vi "Process.vi"(8 "error in":errorcluster, 11 "SMO.EmbeddedUI":refnum<class "Embedded UI.BasicTemplate.lvclass">) -> (0 "error out":errorcluster, 3 "SMO.EmbeddedUI out":refnum<class "Embedded UI.BasicTemplate.lvclass">)   [LabVIEW 2019, in "Embedded UI.BasicTemplate.lvclass"]
doc: "---------------------------------------------------------------\nJKI State Machine Objects™\nhttp://jki.net/state-machine-objects/\nCopyright (C) 2005-2015, JKI <info@jki.net>\nALL RIGHTS RESERVED"
uses:
  Embedded UI.BasicTemplate.lvclass
  C:/Program Files (x86)/National Instruments/LabVIEW 2019/vi.lib/JKI/JKI SMO/SMO/SMO.lvclass
  C:/Users/patrick/Documents/GitHub/Embedded-SMO/lvsrc/SMO.UI.Embedded/SMO.UI.Embedded.lvclass
  <vilib>/JKI/JKI SMO/SMO/Typedefs/Parent Call--Enum.ctl
  <vilib>/JKI/JKI SMO/SMO/SMO.lvclass/SMO.ctl
  Embedded UI/Typedefs/UI State.ctl
  <vilib>/JKI/JKI SMO/SMO/Private/ReftoDVR--SMO.vi
  Embedded UI/Embedded UI.lvclass
  <vilib>/JKI/JKI SMO/SMO/SMO.lvclass
  C:/Users/patrick/Documents/GitHub/Embedded-SMO/lvsrc/SMO.UI.Embedded/Embedded UI.lvclass
  C:/Program Files (x86)/National Instruments/LabVIEW 2019/vi.lib/JKI/JKI SMO/SMO.UI/SMO.UI.lvclass
panel:
  # "Embedded UI SMO\nJoseph Albro,\nLevylab\nUniversity of Pittsburgh\n\nImportant:\nKeep all of the information you want displayed inside this box."
  # "For instructions on how to use the JKI State Machine Objects, examples and video tutorials, visit:\nhttp://jki.net/state-machine-objects/\n\nJKI State Machine Objects™\nhttp://jki.net/state-machine-objects/\nCopyright (C) 2005-2015, JKI <info@jki.net>\nALL RIGHTS RESERVED"
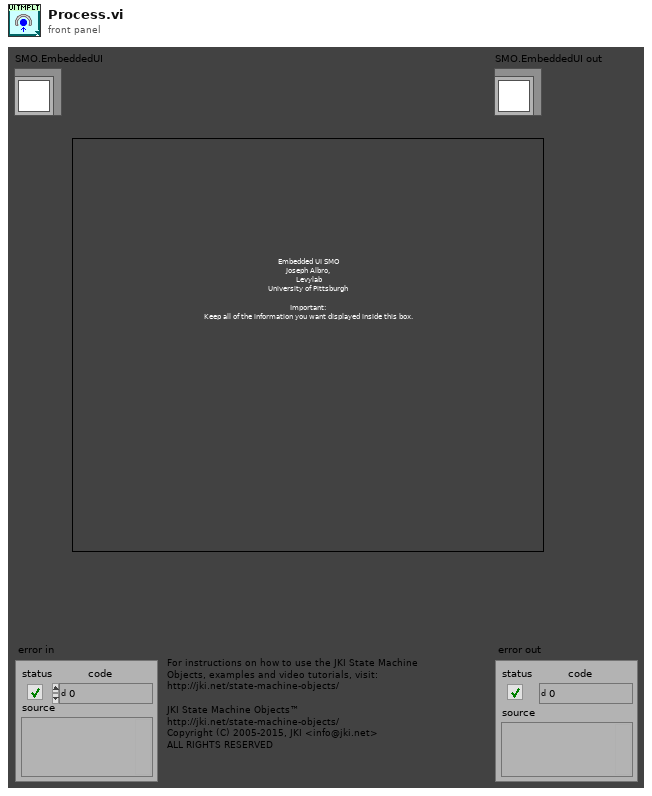
[diagram p1: front panel]
types:
  T1 = typedef "SMO.lvclass/Parent Call--Enum.ctl" = enum16{"Allows parent to run", "Does not request parent to run"}
  T2 = enum32{"invalid app kind", "Development System", "Run Time System", "Student Edition", "Embedded LabVIEW", "Evaluation", "Custom"}
  T3 = enum32{"Invalid", "Standard", "Closed", "Hidden", "Minimized", "Maximized"}
  T4 = enum32{"Bad", "Idle", "Run top level", "Running"}
  T5 = typedef "Embedded UI.lvclass/UI State.ctl" = enum16{"unknown", "Opened", "Embedded", "Closed"}
  T6 = cluster{"Core":cluster{"Current VI Reference":refnum<vi>, "Close Panel on Exit?":bool, "error":errorcluster}, "Self Reference":refnum<class "Embedded UI.BasicTemplate.lvclass">}
  T7 = cluster{"Current VI Reference":refnum<vi>, "Close Panel on Exit?":bool, "error":errorcluster}
  T8 = typedef "SMO.lvclass/Protected Events.ctl" = cluster{"StopProcesses":refnum<user-event>, "AbortProcesses":refnum<user-event>, "Config Changed":refnum<user-event>, "Dependency":refnum<user-event>}
  T9 = typedef "Embedded UI.lvclass/PublicEvents--Cluster.ctl" = cluster{"ReadyForInfo":refnum<user-event>, "UIState":refnum<user-event>}
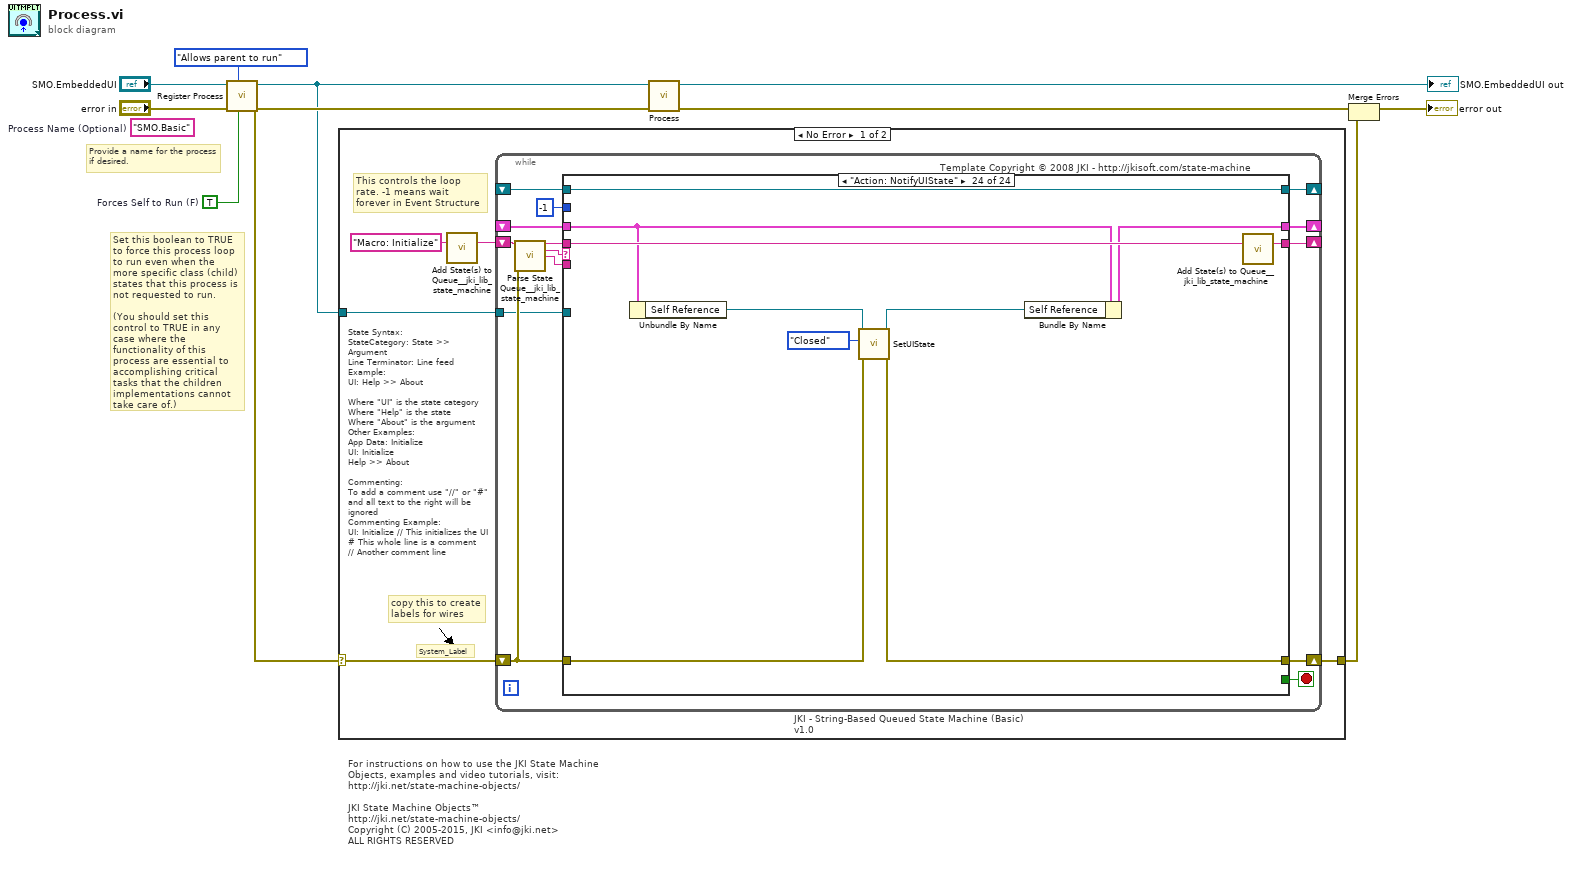
[diagram p0: block diagram]
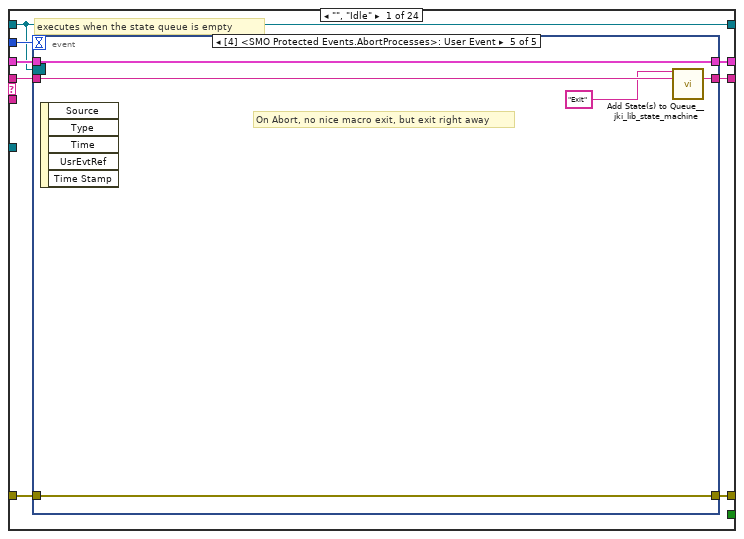
[diagram p2: hidden frame]
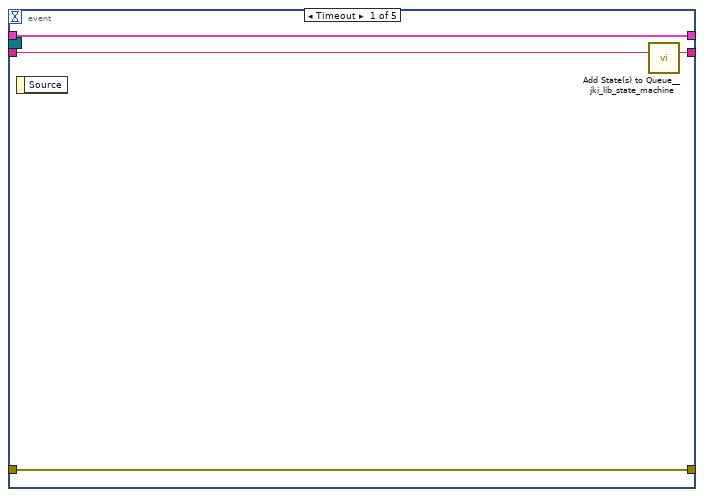
[diagram p3: hidden frame]
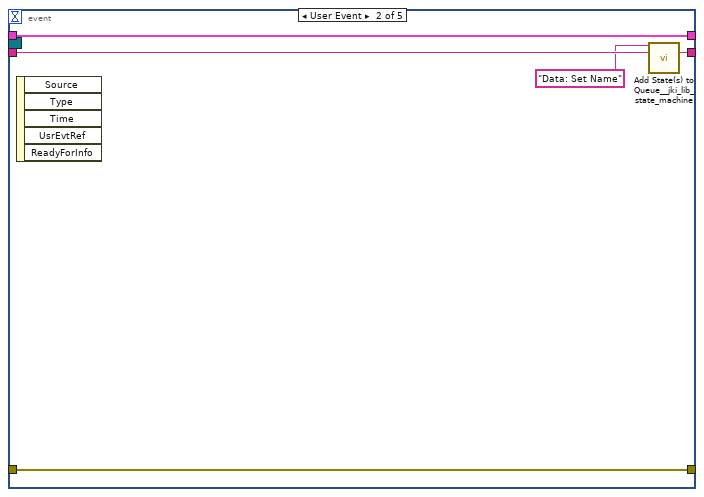
[diagram p4: hidden frame]
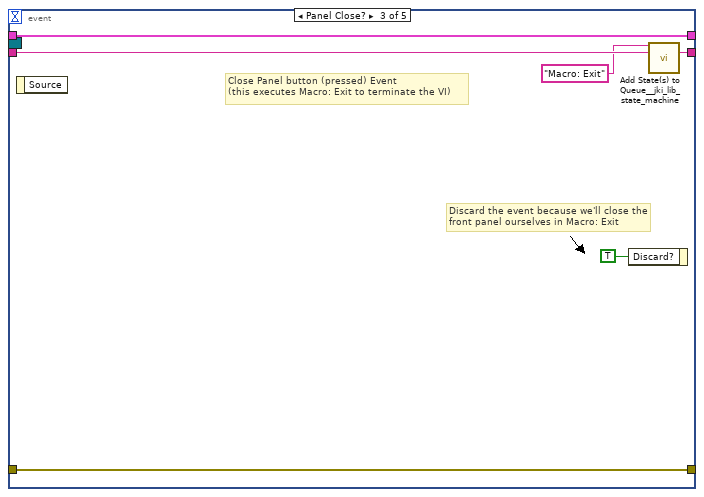
[diagram p5: hidden frame]
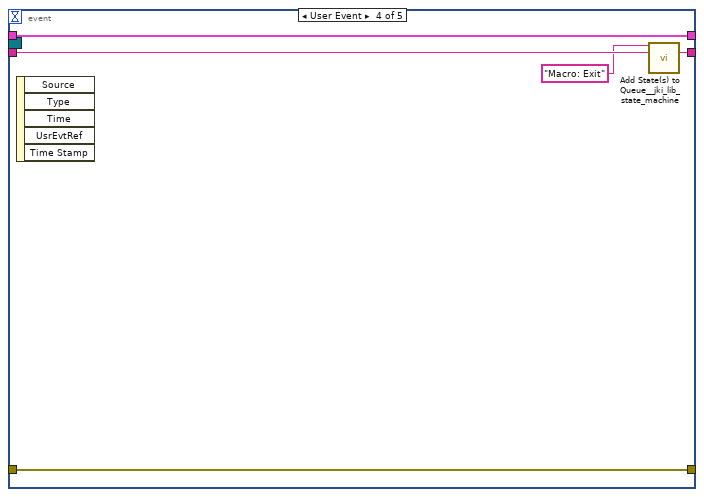
[diagram p6: hidden frame]
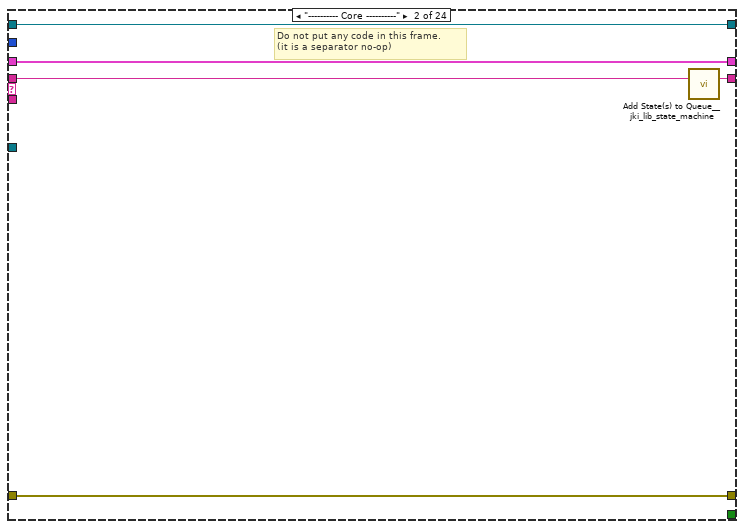
[diagram p7: hidden frame]
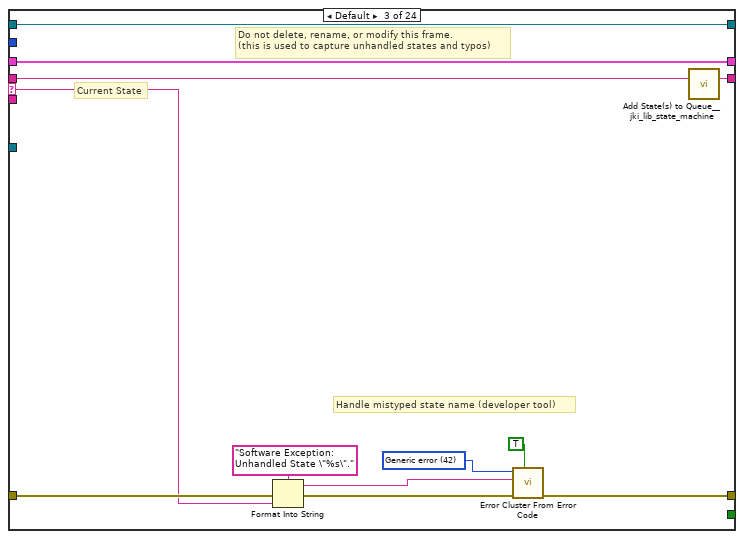
[diagram p8: hidden frame]
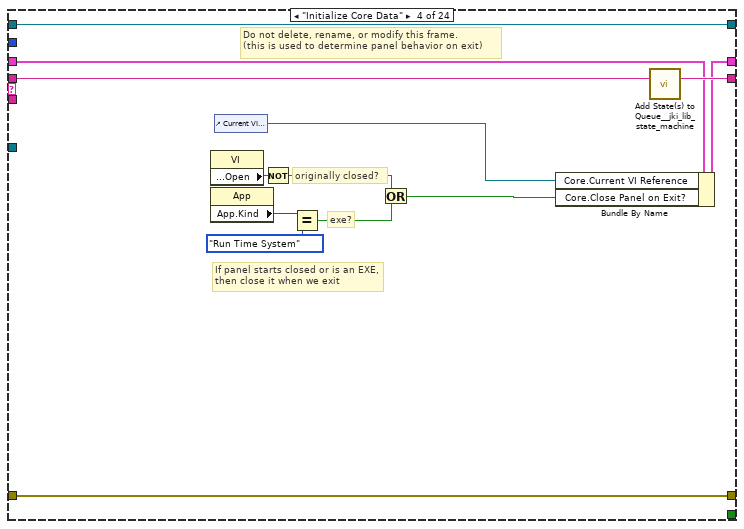
[diagram p9: hidden frame]
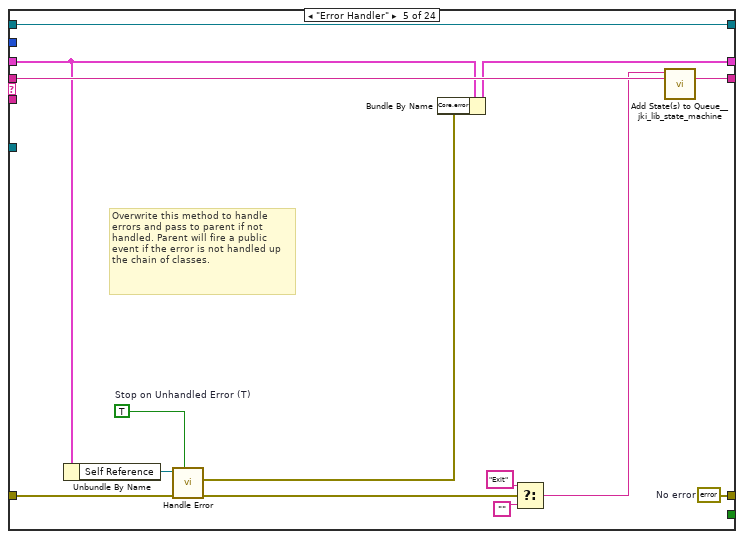
[diagram p10: hidden frame]
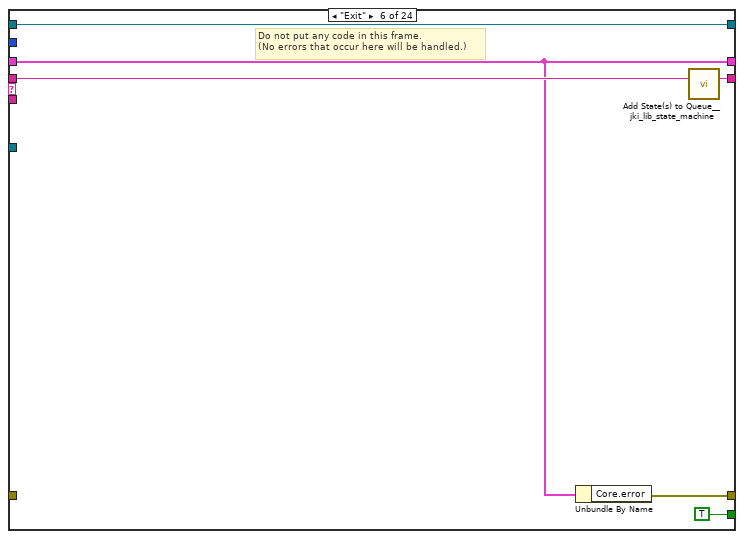
[diagram p11: hidden frame]
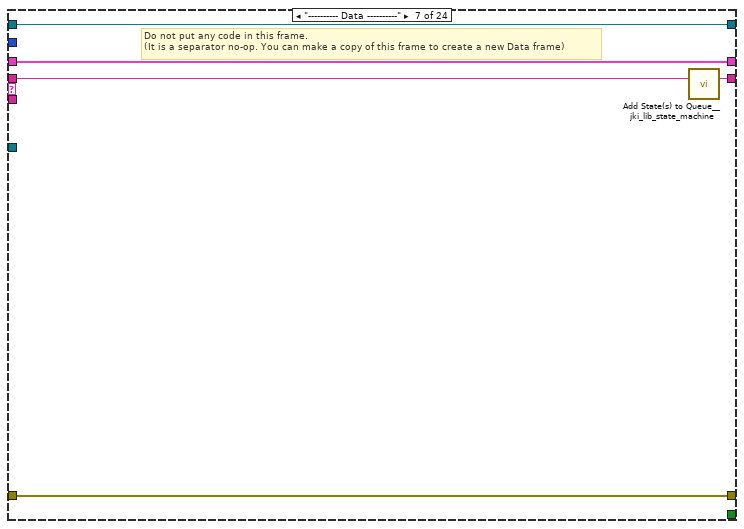
[diagram p12: hidden frame]
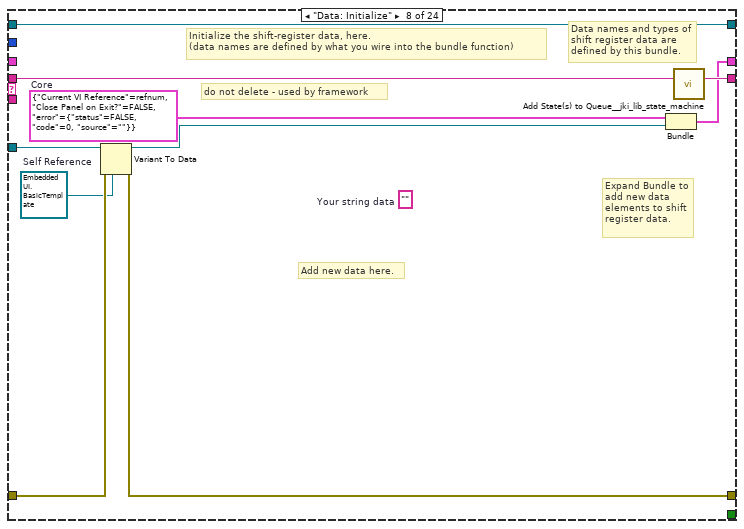
[diagram p13: hidden frame]
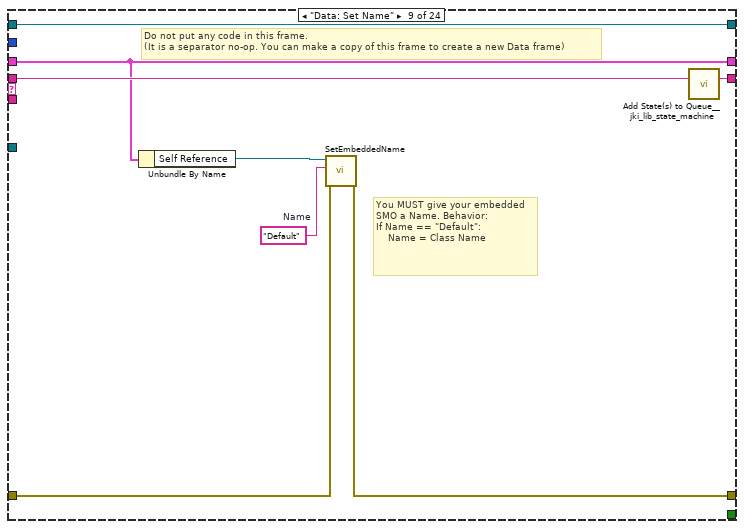
[diagram p14: hidden frame]
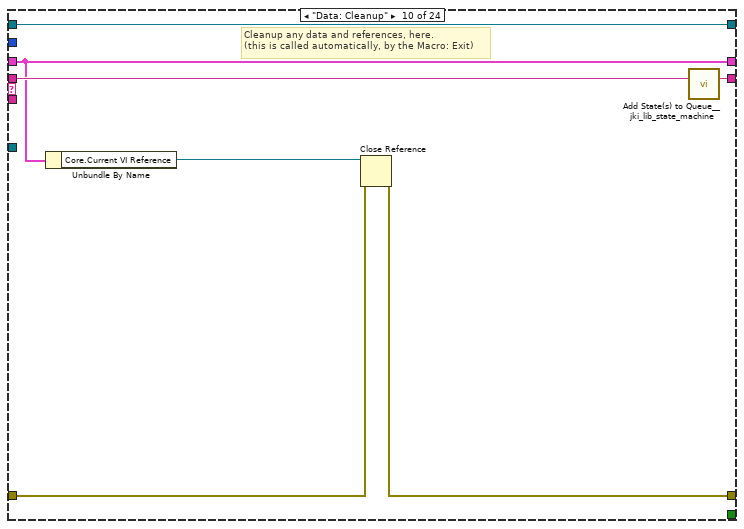
[diagram p15: hidden frame]
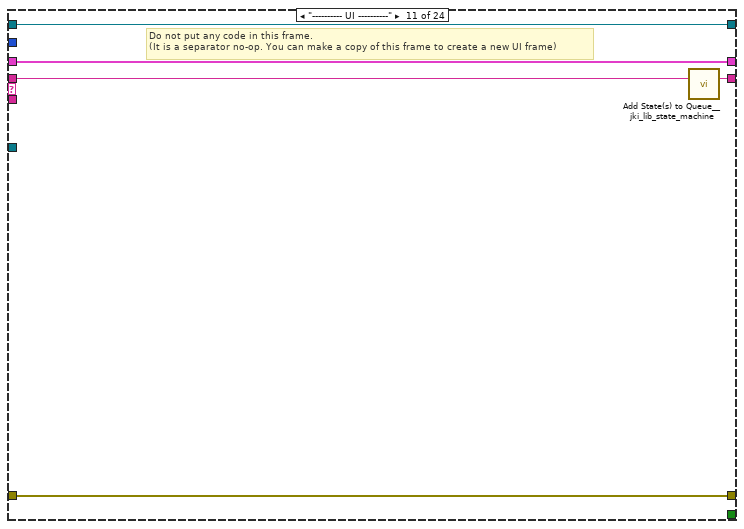
[diagram p16: hidden frame]
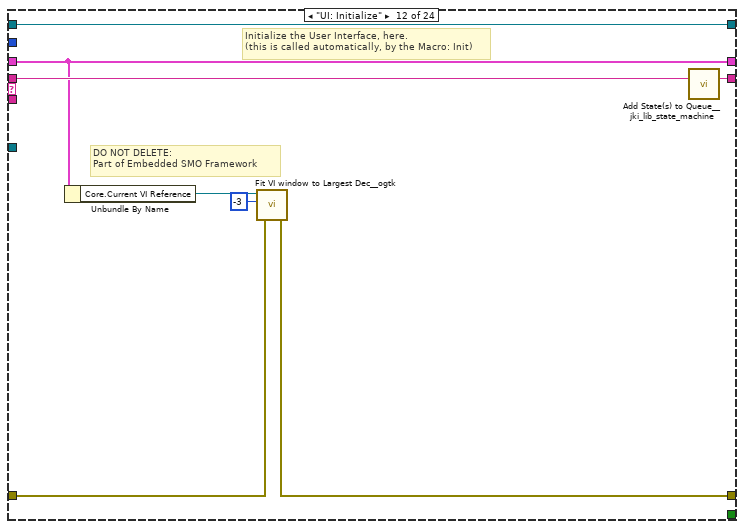
[diagram p17: hidden frame]
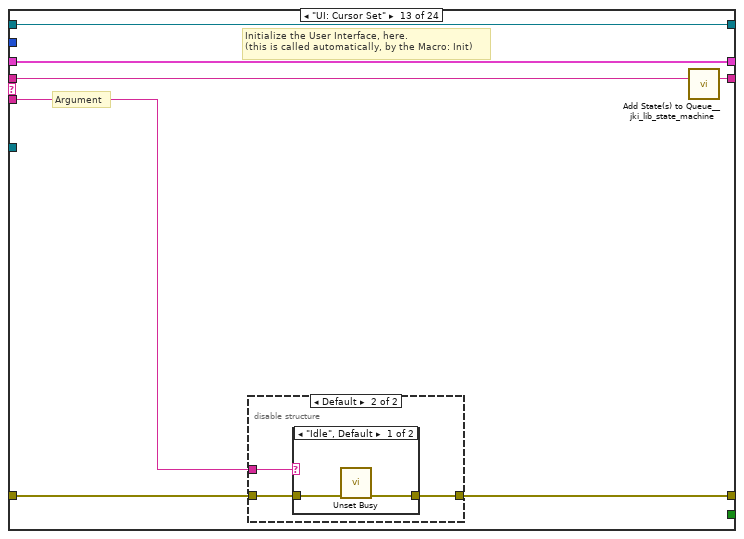
[diagram p18: hidden frame]
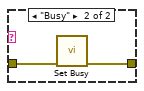
[diagram p20: hidden frame]
diagram:
  w2 = TRUE  # Forces Self to Run (F)
  (unwired) "SMO.Basic"  # Process Name (Optional)
  # "Provide a name for the process\nif desired."
  # "Set this boolean to TRUE to force this process loop to run even when the more specific class (child) states that this process is not requested to run.\n\n(You should set this control to TRUE in any case where the functionality of this process are essential to accomplishing critical tasks that the children implementations cannot take care of.)"
  # "For instructions on how to use the JKI State Machine Objects, examples and video tutorials, visit:\nhttp://jki.net/state-machine-objects/\n\nJKI State Machine Objects™\nhttp://jki.net/state-machine-objects/\nCopyright (C) 2005-2015, JKI <info@jki.net>\nALL RIGHTS RESERVED"
  n1 = call <vilib>:"Register Process.vi"("Forces Self to Run (F)"=w2, "Parent Call"=Parent_Call--Enum."Allows parent to run", "error in (no error)"="error in", "SMO"="SMO.EmbeddedUI") -> ("error out"=w7:errorcluster, "SMO out"=w1:refnum<class "Embedded UI.BasicTemplate.lvclass">)  [unwired: 6 in]
  n2 = case shown="No Error" w7 {
    selector: w7 -> [w12 w293]
    tunnel: w1 -> [w13 _]
    tunnel: [w11 w293] -> w4
    frame No Error {
      # "State Syntax:\nStateCategory: State >> Argument\nLine Terminator: Line feed\nExample:\nUI: Help >> About\n\nWhere \"UI\" is the state category\nWhere \"Help\" is the state\nWhere \"About\" is the argument\nOther Examples:\nApp Data: Initialize\nUI: Initialize\nHelp >> About\n\nCommenting:\nTo add a comment use \"//\" or \"#\" and all text to the right will be ignored\nCommenting Example:\nUI: Initialize // This initializes the UI\n# This whole line is a comment\n// Another comment line"
      # "copy this to create labels for wires"
      # "This controls the loop rate. -1 means wait forever in Event Structure"
      # "System_Label"
      n3 = call <vilib>:"Add State(s) to Queue__jki_lib_state_machine.vi"("State(s) in (\"\")"="Macro: Initialize") -> ("States Out"=w15:string)  [unwired: 14 in]
      n4 = while "JKI - String-Based Queued State Machine (Basic) v1.0" {
        shift-right: [w22] -> _
        shift-left: _ -> [w21]
        shift-right: [w25] -> w11
        shift-left: w12 -> [w19]
        shift-right: [w24] -> _
        shift-left: w15 -> [w26]
        tunnel: w13 -> [w18]
        shift-right: [w17] -> _
        shift-left: _ -> [w16]
        stop <- w23 stop-if-true
        # "Template Copyright © 2008 JKI - http://jkisoft.com/state-machine"
        n5 = call <vilib>:"Parse State Queue__jki_lib_state_machine.vi"("State Queue"=w26, "Error In (no error)"=w19) -> ("Remaining States"=w28:string, "Current State"=w29:string, "Arguments"=w27:string)  [unwired: 11 in]
        n6 = case shown="\"Action: NotifyUIState\"" w29 {
          selector: w29 -> [_ _ w69 _ _ _ _ _ _ _ _ _ _ _ _ _ _ _ _ _ _ _ _ _]
          tunnel: w28 -> [w37 w67 w73 w92 w106 w112 w117 w127 w135 w142 w147 w155 w162 w178 w210 w224 w238 w243 w254 w259 w271 w277 w282 w292]
          tunnel: w27 -> [_ _ _ _ _ _ _ _ _ _ _ _ w156 w172 _ _ _ _ _ _ _ _ _ _]
          tunnel: w21 -> [w35 w64 w71 w83 w100 w108 w114 _ w132 w137 w144 w152 w160 w174 w207 w220 w229 w240 w251 w256 w269 w275 w280 w289]
          tunnel: [w34 w65 w75 w89 w101 w107 w115 w119 w130 w138 w145 w148 w157 w175 w208 w222 w236 w241 w245 w257 w265 w273 w278 w284] -> w25
          tunnel: w19 -> [w33 w65 w74 w89 w102 _ w115 w124 w131 w139 w145 w149 w158 w176 w208 w222 w236 w241 w246 w257 w266 w273 w278 w283]
          tunnel: [w36 w66 w72 w91 w105 w111 w116 w126 w134 w141 w146 w154 w161 w177 w209 w223 w237 w242 w253 w258 w270 w276 w281 w291] -> w24
          tunnel: [_ _ _ _ _ TRUE _ _ _ _ _ _ _ _ _ _ _ _ _ _ _ _ _ _] -> w23
          tunnel: [w32 w64 w71 w90 w99 w108 w114 w125 w132 w137 w144 w152 w160 w174 w207 w220 w229 w240 w251 w256 w269 w275 w280 w288] -> w22
          tunnel: -1 ("Timeout") -> [w31 _ _ _ _ _ _ _ _ _ _ _ _ _ _ _ _ _ _ _ _ _ _ _]
          tunnel: w18 -> [_ _ _ _ _ _ _ w122 _ _ _ _ _ _ _ _ _ _ _ _ _ _ _ _]
          tunnel: [w30 w63 w68 w80 w104 w109 w113 w121 w133 w136 w143 w153 w159 w171 w206 w221 w230 w239 w252 w255 w268 w274 w279 w290] -> w17
          tunnel: w16 -> [w30 w63 w68 w80 w104 w109 w113 w121 w133 w136 w143 w153 w159 w171 w206 w221 w230 w239 w252 w255 _ w274 w279 w290]
          frame "", "Idle" {
            # "executes when the state queue is empty"
            n7 = event shown="[4] <SMO Protected Events.AbortProcesses>: User Event" {
              selector: w30 -> [_ _ _ _ _]
              dyn-events: _ -> [_ _ _ _ _]
              timeout: w31 -> [_ _ _ _ _]
              tunnel: w37 -> [w41 w46 w52 w57 w62]
              tunnel: [w40 w45 w51 w56 w61] -> w36
              tunnel: w35 -> [w39 w44 w49 w54 w59]
              tunnel: [w38 w43 w50 w55 w60] -> w34
              tunnel: w33 -> [w38 w43 w50 w55 w60]
              tunnel: [w39 w44 w49 w54 w59] -> w32
              event Timeout {
                n8 = event-data() -> ()  [unwired: 1 in, 1 out]
                n9 = call <vilib>:"Add State(s) to Queue__jki_lib_state_machine.vi"("State(s) in (\"\")"=w41) -> ("States Out"=w40:string)  [unwired: 14 in]
              }
              event User Event {
                n10 = event-data() -> ()  [unwired: 1 in, 5 out]
                n11 = call <vilib>:"Add State(s) to Queue__jki_lib_state_machine.vi"("State(s) in Front (\"\")"="Data: Set Name" ("State(s) in Front (\"\")"), "State(s) in (\"\")"=w46) -> ("States Out"=w45:string)  [unwired: 13 in]
              }
              event Panel Close? {
                # "Discard the event because we'll close the front panel ourselves in Macro: Exit"
                # "Close Panel button (pressed) Event\n(this executes Macro: Exit to terminate the VI)"
                n12 = event-data() -> ()  [unwired: 1 in, 1 out]
                n13 = event-data("Discard?"=TRUE) -> ()  [unwired: 1 in, 1 out]
                n14 = call <vilib>:"Add State(s) to Queue__jki_lib_state_machine.vi"("State(s) in Front (\"\")"="Macro: Exit", "State(s) in (\"\")"=w52) -> ("States Out"=w51:string)  [unwired: 13 in]
              }
              event User Event {
                n15 = event-data() -> ()  [unwired: 1 in, 5 out]
                n16 = call <vilib>:"Add State(s) to Queue__jki_lib_state_machine.vi"("State(s) in Front (\"\")"="Macro: Exit", "State(s) in (\"\")"=w57) -> ("States Out"=w56:string)  [unwired: 13 in]
              }
              event User Event {
                # "On Abort, no nice macro exit, but exit right away"
                n17 = event-data() -> ()  [unwired: 1 in, 5 out]
                n18 = call <vilib>:"Add State(s) to Queue__jki_lib_state_machine.vi"("State(s) in Front (\"\")"="Exit", "State(s) in (\"\")"=w62) -> ("States Out"=w61:string)  [unwired: 13 in]
              }
            }
          }
          frame "---------- Core ----------" {
            # "Do not put any code in this frame.\n(it is a separator no-op)"
            n19 = call <vilib>:"Add State(s) to Queue__jki_lib_state_machine.vi"("State(s) in (\"\")"=w67) -> ("States Out"=w66:string)  [unwired: 14 in]
          }
          frame Default {
            w78 = 42 items=["No error", "Argument error", "Memory is full", "Out of zone", "End of file", "File already open", "Generic file I/O error", "File not found", "File permission error", "Disk is full", "Duplicate path", "Too many files open", "System feature not enabled", "Resource file not found", "Cannot add resource", "Resource not found", "Image not found", "Image memory error", "Pen does not exist", "Config type invalid", "Config token not found", "Config parse error", "Config memory error", "Bad external code format", "Bad external code offset", "External code not present", "Null window", "Destroy window error", "Null menu", "Print aborted", "Bad print record", "Print driver error", "Windows error during printing", "Memory error during printing", "Print dialog error", "Generic print error", "Invalid device refnum", "Device not found", "Device parameter error", "Device unit error", "Cannot open device", "Device call aborted", "Generic error", "Cancelled by user", "Object ID too low", "Object ID too high", "Object not in heap", "Unknown heap", "Unknown object (invalid DefProc)", "Unknown object (DefProc not in table)", "Message out of range", "Invalid (null) method", "Unknown message", "Manager call not supported", "Bad address", "Network operation in progress", "Network operation timed out", "Connection is busy", "Network attribute not supported", "Network error", "Address in use", "System out of memory", "Connection aborted", "Connection refused", "Not connected", "Already connected", "Connection closed", "Initialization error (interapplication manager)", "Bad occurrence", "Wait on unbound occurrence handler", "Occurrence queue overflow", "Datalog type conflict", "Unused", "Unrecognized type (interapplication manager)", "Memory corrupt", "Failed to make temporary DLL", "Old CIN version", "Drag socket not found", "Failed to load drop-object", "Failed to register OLE object", "Failed to release OLE object", "Format specifier type mismatch", "Unknown format specifier", "Too few format specifiers", "Too many format specifiers", "Scan failed", "Newer CIN version", "Error converting to variant", "Runtime menu error", "Password tampered", "Variant attribute not found", "Incompatible variant data type", "Event data is not available", "Event Store is not present", "Occurrence is not found", "Event Queue is not created", "Event info is not available", "Refnum passed is NULL", "Error retrieving Class GUID", "Error retrieving CoClass GUID", "Error retrieving TypeLib GUID.", "Bad built application magic bytes.", "Specific driver is different from the specific driver associated with the Logical Name.", "There is no session opened to the class driver.", "Max Error", "MAX - Error with config objects", "MAX - Error loading configuration", "MAX - Group not supported"]
            # "Current State"
            # "Do not delete, rename, or modify this frame.\n(this is used to capture unhandled states and typos)"
            # "Handle mistyped state name (developer tool)"
            n20 = Format Into String(format string="Software Exception: Unhandled State \"%s\"." ("message"), error in=w74, w69) -> (resulting string=w77:string, error out=w76:errorcluster)  [unwired: 1 in]
            n21 = call <vilib>:"Error Cluster From Error Code.vi"("show call chain? (False)"=TRUE, "error in (no error)"=w76, "error message (\"\")"=w77, "error code (0)"=w78) -> ("error out"=w75:errorcluster)  [unwired: 5 in]
            n22 = call <vilib>:"Add State(s) to Queue__jki_lib_state_machine.vi"("State(s) in (\"\")"=w73) -> ("States Out"=w72:string)  [unwired: 14 in]
          }
          frame "Initialize Core Data" {
            # "Do not delete, rename, or modify this frame.\n(this is used to determine panel behavior on exit)"
            # "originally closed?"
            # "exe?"
            # "If panel starts closed or is an EXE, then close it when we exit"
            n23 = property class="VI"() -> ("Front Panel.Open"=w88:bool)  [unwired: 2 in, 2 out]
            n24 = property class="App"() -> ("App.Kind"=w87:T2)  [unwired: 2 in, 2 out]
            n25 = control-ref of="Current VI Reference"() -> (w81:refnum<vi>)
            n26 = Not(x=w88) -> (.not. x?=w85:bool)
            n27 = Equal?(x=w87, y=T2."Run Time System" ("Application:Kind")) -> (x = y?=w84:bool)
            n28 = Or(x=w85, y=w84) -> (x .or. y?=w82:bool)
            n29 = Bundle By Name(cluster=w83, "Core.Current VI Reference"=w81, "Core.Close Panel on Exit?"=w82) -> (w90:T6)
            n30 = call <vilib>:"Add State(s) to Queue__jki_lib_state_machine.vi"("State(s) in (\"\")"=w92) -> ("States Out"=w91:string)  [unwired: 14 in]
          }
          frame "Error Handler" {
            w93 = TRUE  # Stop on Unhandled Error (T)
            w101 = errorcluster {"status"=FALSE, "code"=0, "source"=""}  # No error
            # "Overwrite this method to handle errors and pass to parent if not handled. Parent will fire a public event if the error is not handled up the chain of classes."
            n31 = Unbundle By Name(w100) -> ("Self Reference"=w103:refnum<class "Embedded UI.BasicTemplate.lvclass">)
            n32 = call-dynamic "Handle Error.vi"("Stop on Unhandled Error (T)"=w93, "error in"=w102, "SMO"=w103) -> ("handling error"=w94:errorcluster, "Unhandled error"=w97:errorcluster)  [unwired: 6 in, 1 out]
            n33 = Bundle By Name(cluster=w100, "Core.error"=w97) -> (w99:T6)
            n34 = Select(t="Exit", s=w94, f="") -> (s? t:f=w98:string)
            n35 = call <vilib>:"Add State(s) to Queue__jki_lib_state_machine.vi"("State(s) in Front (\"\")"=w98, "State(s) in (\"\")"=w106) -> ("States Out"=w105:string)  [unwired: 13 in]
          }
          frame "Exit" {
            # "Do not put any code in this frame.\n(No errors that occur here will be handled.)"
            n36 = Unbundle By Name(w108) -> ("Core.error"=w107:errorcluster)
            n37 = call <vilib>:"Add State(s) to Queue__jki_lib_state_machine.vi"("State(s) in (\"\")"=w112) -> ("States Out"=w111:string)  [unwired: 14 in]
          }
          frame "---------- Data ----------" {
            # "Do not put any code in this frame.\n(It is a separator no-op. You can make a copy of this frame to create a new Data frame)"
            n38 = call <vilib>:"Add State(s) to Queue__jki_lib_state_machine.vi"("State(s) in (\"\")"=w117) -> ("States Out"=w116:string)  [unwired: 14 in]
          }
          frame "Data: Initialize" {
            w120 = T7 {"Current VI Reference"=refnum, "Close Panel on Exit?"=FALSE, "error"={"status"=FALSE, "code"=0, "source"=""}}  # Core
            w123 = refnum<class "Embedded UI.BasicTemplate.lvclass"> refnum  # Self Reference
            (unwired) ""  # Your string data
            # "do not delete - used by framework"
            # "Expand Bundle to add new data elements to shift register data."
            # "Add new data here."
            # "Data names and types of shift register data are defined by this bundle."
            # "Initialize the shift-register data, here.\n(data names are defined by what you wire into the bundle function)"
            n39 = Variant To Data(error in=w124, type=w123, Variant=w122) -> (data=w118:refnum<class "Embedded UI.BasicTemplate.lvclass">, error out=w119:errorcluster)
            n40 = Bundle("Core"=w120, "Self Reference"=w118) -> (w125:T6)  [unwired: 1 in]
            n41 = call <vilib>:"Add State(s) to Queue__jki_lib_state_machine.vi"("State(s) in (\"\")"=w127) -> ("States Out"=w126:string)  [unwired: 14 in]
          }
          frame "Data: Set Name" {
            w129 = "Default"  # Name
            # "You MUST give your embedded SMO a Name. Behavior:\nIf Name == \"Default\":\n    Name = Class Name"
            # "Do not put any code in this frame.\n(It is a separator no-op. You can make a copy of this frame to create a new Data frame)"
            n42 = Unbundle By Name(w132) -> ("Self Reference"=w128:refnum<class "Embedded UI.BasicTemplate.lvclass">)
            n43 = call "SetEmbeddedName.vi"("error in (no error)"=w131, "Name"=w129, "EmbeddedSMO in"=w128) -> ("error out"=w130:errorcluster)  [unwired: 7 in, 1 out]
            n44 = call <vilib>:"Add State(s) to Queue__jki_lib_state_machine.vi"("State(s) in (\"\")"=w135) -> ("States Out"=w134:string)  [unwired: 14 in]
          }
          frame "Data: Cleanup" {
            # "Cleanup any data and references, here.\n(this is called automatically, by the Macro: Exit)"
            n45 = Unbundle By Name(w137) -> ("Core.Current VI Reference"=w140:refnum<vi>)
            n46 = Close Reference(reference=w140, error in (no error)=w139) -> (error out=w138:errorcluster)
            n47 = call <vilib>:"Add State(s) to Queue__jki_lib_state_machine.vi"("State(s) in (\"\")"=w142) -> ("States Out"=w141:string)  [unwired: 14 in]
          }
          frame "---------- UI ----------" {
            # "Do not put any code in this frame.\n(It is a separator no-op. You can make a copy of this frame to create a new UI frame)"
            n48 = call <vilib>:"Add State(s) to Queue__jki_lib_state_machine.vi"("State(s) in (\"\")"=w147) -> ("States Out"=w146:string)  [unwired: 14 in]
          }
          frame "UI: Initialize" {
            # "DO NOT DELETE:\nPart of Embedded SMO Framework"
            # "Initialize the User Interface, here.\n(this is called automatically, by the Macro: Init)"
            n49 = Unbundle By Name(w152) -> ("Core.Current VI Reference"=w151:refnum<vi>)
            n50 = call <userlib>:"Fit VI window to Largest Dec__ogtk.vi"("error in (no error)"=w149, "border spacing (2 px)"=-3, "VI Ref (calling VI)"=w151) -> ("error out"=w148:errorcluster)  [unwired: 3 in, 1 out]
            n51 = call <vilib>:"Add State(s) to Queue__jki_lib_state_machine.vi"("State(s) in (\"\")"=w155) -> ("States Out"=w154:string)  [unwired: 14 in]
          }
          frame "UI: Cursor Set" {
            # "Argument"
            # "Initialize the User Interface, here.\n(this is called automatically, by the Macro: Init)"
            n52 = disable-structure shown="Default" {
              disable-tunnel: w158 -> [w163 w166]
              disable-tunnel: [w163 w165] -> w157
              disable-tunnel: w156 -> [_ w164]
              frame condition #0 {
              }
              frame condition #1 (active) {
                n53 = case shown="\"Idle\", Default" w164 {
                  tunnel: w166 -> [w168 w170]
                  tunnel: [w167 w169] -> w165
                  frame "Idle", Default {
                    n54 = call <vilib>:"Unset Busy.vi"("error in (no error)"=w168) -> ("error out"=w167:errorcluster)  [unwired: 10 in]
                  }
                  frame "Busy" {
                    n55 = call <vilib>:"Set Busy.vi"("error in (no error)"=w170) -> ("error out"=w169:errorcluster)  [unwired: 9 in, 1 out]
                  }
                }
              }
            }
            n56 = call <vilib>:"Add State(s) to Queue__jki_lib_state_machine.vi"("State(s) in (\"\")"=w162) -> ("States Out"=w161:string)  [unwired: 14 in]
          }
          frame "UI: Front Panel State" {
            # "Argument"
            # "Set Front Panel Open or Closed\n(Usage: \"UI: Front Panel State >> Open|Close\")"
            n57 = Unbundle By Name(w174) -> ("Core.Current VI Reference"=w173:refnum<vi>)
            n58 = disable-structure shown="Default" {
              disable-tunnel: w176 -> [w182 w205]
              disable-tunnel: [w181 w205] -> w175
              disable-tunnel: w173 -> [w180 _]
              disable-tunnel: w172 -> [w179 _]
              frame condition #0 (active) {
                n59 = case shown="\"Close\"" w179 {
                  tunnel: w182 -> [w186 w199]
                  tunnel: [w188 w200] -> w181
                  tunnel: w180 -> [w187 w197]
                  frame "Open", Default {
                    n60 = property class="VI"(reference=w187, error in=w186) -> (reference out=w184:refnum<vi>, error out=w185:errorcluster, "FP.State"=w183:T3)
                    n61 = case shown="\"Closed\"" w183 {
                      tunnel: [w191 w194] -> w188
                      tunnel: w185 -> [w190 w194]
                      tunnel: w184 -> [w189 _]
                      frame "Closed" {
                        n62 = invoke class="VI" method="FP.Open"(reference=w189, error in=w190, "Activate"=TRUE, "State"=T3."Standard") -> (error out=w191:errorcluster)  [unwired: 1 in, 4 out]
                      }
                      frame Default {
                      }
                    }
                  }
                  frame "Close" {
                    n63 = property class="VI"(reference=w197, error in=w199) -> (reference out=w196:refnum<vi>, error out=w198:errorcluster, "FP.State"=w195:T3)
                    n64 = case shown="Default" w195 {
                      tunnel: [w201 w204] -> w200
                      tunnel: w198 -> [w201 w203]
                      tunnel: w196 -> [_ w202]
                      frame "Invalid", "Closed" {
                      }
                      frame Default {
                        n65 = invoke class="VI" method="FP.Close"(reference=w202, error in=w203) -> (error out=w204:errorcluster)  [unwired: 1 in, 2 out]
                      }
                    }
                  }
                }
              }
              frame condition #1 {
              }
            }
            n66 = call <vilib>:"Add State(s) to Queue__jki_lib_state_machine.vi"("State(s) in (\"\")"=w178) -> ("States Out"=w177:string)  [unwired: 14 in]
          }
          frame "---------- Macro ----------" {
            # "Do not put any code in this frame.\n(It is a separator no-op. You can make a copy of this frame to create a new Macro frame)"
            n67 = call <vilib>:"Add State(s) to Queue__jki_lib_state_machine.vi"("State(s) in (\"\")"=w210) -> ("States Out"=w209:string)  [unwired: 14 in]
          }
          frame "Macro: Initialize" {
            w215 = "UI: Initialize\nData: Set Name\n//UI: Front Panel State >> Open"  # UI: Initialize Data: Set Name //UI: Front Panel State >> Open
            w211 = "Process: Sync"
            # "Initialization Macro\n(This is called once, when the VI starts)"
            n68 = control-ref of="This VI"() -> (w213:refnum<vi>)
            n69 = property class="VI"(reference=w213) -> ("Exec.State"=w212:T4)  [unwired: 1 in, 2 out]
            n70 = Equal?(x=w212, y=T4."Run top level") -> (x = y?=w218:bool)
            n71 = Select(t=w211, s=w218, f="") -> ()  [unwired: 1 out]
            n72 = call <vilib>:"Add State(s) to Queue__jki_lib_state_machine.vi"("State(s) in Front (\"\")"="Data: Initialize\nInitialize Core Data\nEvents: Register", "State(s) in (\"\")"=w211, "State(s) at Back (\"\")"=w215) -> ("States Out"=w214:string)  [unwired: 12 in]
            n73 = call <vilib>:"Add State(s) to Queue__jki_lib_state_machine.vi"("State(s) in Front (\"\")"=w214, "State(s) in (\"\")"=w224) -> ("States Out"=w223:string)  [unwired: 13 in]
          }
          frame "Macro: Exit" {
            # "Exit Macro\n(This is called once, when the VI exits)"
            n74 = Unbundle By Name(w229) -> ("Core.Close Panel on Exit?"=w235:bool)
            n75 = Select(t="UI: Front Panel State >> Close\nAction: NotifyUIState", s=w235, f="") -> (s? t:f=w232:string)
            n76 = call <vilib>:"Add State(s) to Queue__jki_lib_state_machine.vi"("State(s) in Front (\"\")"="Data: Cleanup\nEvents: Unregister", "State(s) in (\"\")"="Process: Sync", "State(s) at Back (\"\")"="Exit") -> ("States Out"=w226:string)  [unwired: 12 in]
            n77 = call <vilib>:"Add State(s) to Queue__jki_lib_state_machine.vi"("State(s) in (\"\")"=w232, "State(s) at Back (\"\")"=w226) -> ("States Out"=w231:string)  [unwired: 13 in]
            n78 = call <vilib>:"Add State(s) to Queue__jki_lib_state_machine.vi"("State(s) in Front (\"\")"=w231, "State(s) in (\"\")"=w238) -> ("States Out"=w237:string)  [unwired: 13 in]
          }
          frame "---------- Process ----------" {
            # "Template Separator\n(You can make a copy of, or modify, this frame)"
            n79 = call <vilib>:"Add State(s) to Queue__jki_lib_state_machine.vi"("State(s) in (\"\")"=w243) -> ("States Out"=w242:string)  [unwired: 14 in]
          }
          frame "Process: Sync" {
            n80 = Unbundle By Name(w251) -> ("Self Reference"=w247:refnum<class "Embedded UI.BasicTemplate.lvclass">)
            n81 = call <vilib>:"WaitOnProcessSync.vi"("error in (no error)"=w246, "SMO"=w247) -> ("error out"=w245:errorcluster, "Don't run?"=w250:bool)  [unwired: 7 in, 1 out]
            n82 = Select(t="Data: Cleanup\nEvents: Unregister\nExit", s=w250, f="") -> (s? t:f=w244:string)
            n83 = call <vilib>:"Add State(s) to Queue__jki_lib_state_machine.vi"("State(s) in Front (\"\")"=w244, "State(s) in (\"\")"=w254) -> ("States Out"=w253:string)  [unwired: 13 in]
          }
          frame "---------- Events ----------" {
            # "Template Separator\n(You can make a copy of, or modify, this frame)"
            n84 = call <vilib>:"Add State(s) to Queue__jki_lib_state_machine.vi"("State(s) in (\"\")"=w259) -> ("States Out"=w258:string)  [unwired: 14 in]
          }
          frame "Events: Register" {
            # "Expand to add\nmore events"
            n85 = Unbundle By Name(w269) -> ("Self Reference"=w260:refnum<class "Embedded UI.BasicTemplate.lvclass">)
            n86 = call <vilib>:"GetProtectedEvents.vi"("SMO"=w260) -> ("error out"=w263:errorcluster, "SMO Protected Events"=w267:T8)  [unwired: 8 in, 1 out]
            n87 = call "Embedded UI.GetPublicEvents.vi"("EmbeddedSMO"=w260) -> ("error out"=w261:errorcluster, "Public Events"=w262:T9)  [unwired: 8 in, 1 out]
            n88 = register-events(w267, w262) -> (reference out=w268:refnum<event-registration>, error out=w264:errorcluster)  [unwired: 2 in]
            n89 = Merge Errors(w266, w264, w263, w261) -> (w265:errorcluster)
            n90 = call <vilib>:"Add State(s) to Queue__jki_lib_state_machine.vi"("State(s) in (\"\")"=w271) -> ("States Out"=w270:string)  [unwired: 14 in]
          }
          frame "Events: Unregister" {
            n91 = Unregister For Events(event registration refnum=w274, error in=w273) -> (error out=w272:errorcluster)
            n92 = call <vilib>:"Clear Errors.vi"("error in (no error)"=w272) -> ()  [unwired: 5 in, 2 out]
            n93 = call <vilib>:"Add State(s) to Queue__jki_lib_state_machine.vi"("State(s) in (\"\")"=w277) -> ("States Out"=w276:string)  [unwired: 14 in]
          }
          frame "---------- Action ----------" {
            n94 = call <vilib>:"Add State(s) to Queue__jki_lib_state_machine.vi"("State(s) in (\"\")"=w282) -> ("States Out"=w281:string)  [unwired: 14 in]
          }
          frame "Action: NotifyUIState" {
            n95 = Unbundle By Name(w289) -> ("Self Reference"=w287:refnum<class "Embedded UI.BasicTemplate.lvclass">)
            n96 = call "SetUIState.vi"("error in (no error)"=w283, "UI State"=UI_State."Closed", "EmbeddedSMO in"=w287) -> ("error out"=w284:errorcluster, "EmbeddedSMO out"=w286:refnum<class "Embedded UI.BasicTemplate.lvclass">)  [unwired: 7 in]
            n97 = Bundle By Name(cluster=w289, "Self Reference"=w286) -> (w288:T6)
            n98 = call <vilib>:"Add State(s) to Queue__jki_lib_state_machine.vi"("State(s) in (\"\")"=w292) -> ("States Out"=w291:string)  [unwired: 14 in]
          }
        }
      }
    }
    frame Error {
    }
  }
  n99 = call-parent "Process.vi"("error in"=w7, "EmbeddedSMO"=w1) -> ("error out"=w5:errorcluster, "EmbeddedSMO out"=→"SMO.EmbeddedUI out":refnum<class "Embedded UI.BasicTemplate.lvclass">)  [unwired: 8 in]
  n100 = Merge Errors(w5, w4) -> (→"error out":errorcluster)
